vi "XCtrl-State Changed.vi"(10 "Action":T1 caption="Action In") -> (2 "Action 2":T1 caption="Action Out")   [LabVIEW 2012]
doc: "This is a handy utility VI created to be used with XControls. It isn't part of the XControl since it is used in several places. It updates the setting of the State Changed boolean"
uses:
  <vilib>/_xctls/Action.ctl
  <vilib>/_xctls/XControlSupport.lvlib
panel:
  # "Overview: This is a handy utility VI created to be used with XControls. It isn't part of the XControl since it is used in several places. It updates the setting of the State Changed boolean"
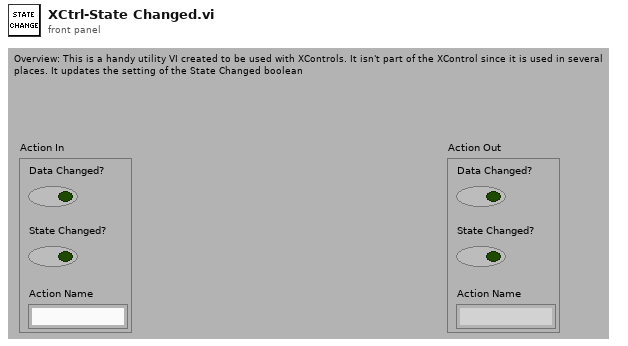
[diagram p1: front panel]
types:
  T1 = typedef "XControlSupport.lvlib/Action.ctl" = cluster{"Data Changed?":bool, "State Changed?":bool, "Action Name":string}
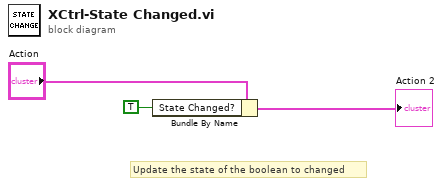
[diagram p0: block diagram]
diagram:
  # "Update the state of the boolean to changed"
  n1 = Bundle By Name(cluster="Action", "State Changed?"=TRUE) -> (→"Action 2":T1)
